vi "Frames.Initialize.vi"(6 "Direction":T1(ring), 8 "error in":errorcluster, 9 "Lookup":variant, 10 "Frames":T2[](array[typedef]) {"Signals"."Byte Order" items=["Little Endian", "Big Endian"]; "Signals"."Data Type" items=["Signed", "Unsigned", "IEEE Float"]}, 11 "Cluster In":refnum<k21>) -> (0 "error out":errorcluster, 1 "Lookup":variant, 3 "Cluster Out":refnum<k21>)   [LabVIEW 2019, in "Diagnostics Addon Engine.lvlib"]
uses:
  Diagnostics Addon Engine.lvlib
  Addon Shared/Types/Frame.Compile.ctl
  Addon Shared/Types/Type.ctl
  Addon Shared/Types/Signal.ctl
  Addon Shared/Types/XNET.Frame.ctl
  Addon Shared/SubVIs/Constants.vi
  <vilib>/xnet/xnet.llb/XNET Create Session (Conversion).vi
  Addon Shared/Diagnostics Addon Shared.lvlib
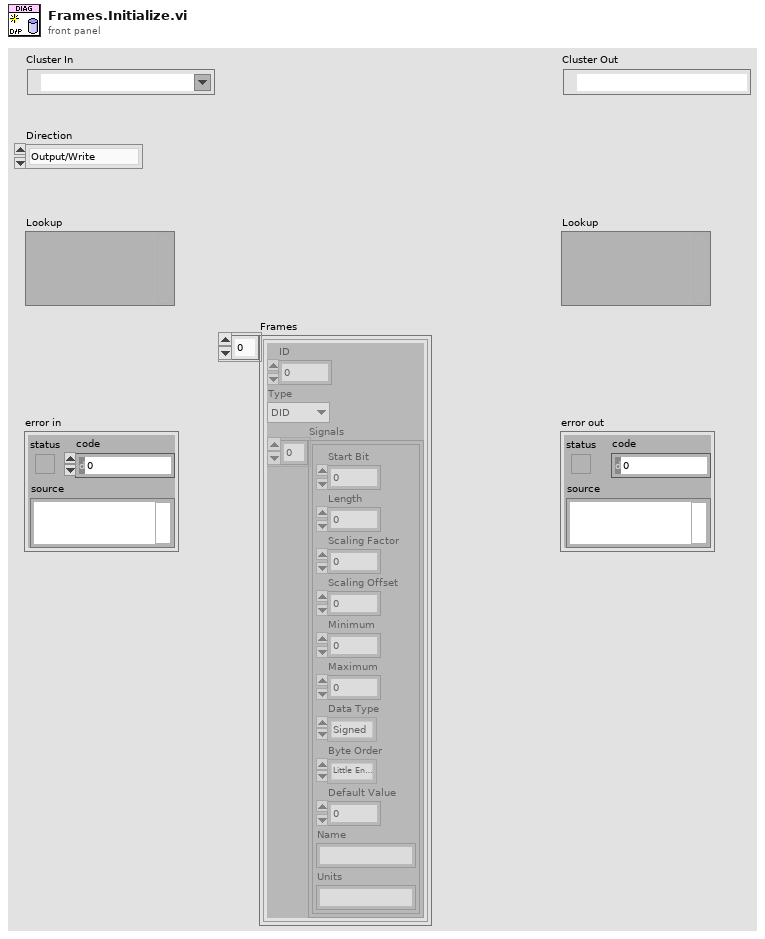
[diagram p1: front panel]
types:
  T1 = enum16{"Output/Write", "Input/Read", "Input/ReadWrite"}
  T2 = typedef "Diagnostics Addon Shared.lvlib/Frame.Compile.ctl" = cluster{"ID":u32, "Type":T3, "Signals":T4[]}
  T3 = typedef "Diagnostics Addon Shared.lvlib/Type.ctl" = enum16{"DID", "CDID", "PID", "CPID", "Read Memory", "Write Memory", "IO Control", "Routine Start", "Routine Request", "Routine Stop", "User Defined", "DTC Control", "Clear DTCs", "Read DTCs", "Start DTCs", "DTC Change Count", "Tester Present", "Unlock ECU", "Reset ECU", "Diag Session Control", "Communication Control", "DPID Control", "Poll Control", "Diag CAN Control"}
  T4 = typedef "Diagnostics Addon Shared.lvlib/Signal.ctl" = cluster{"Start Bit":u32, "Length":u32, "Scaling Factor":dbl, "Scaling Offset":dbl, "Minimum":dbl, "Maximum":dbl, "Data Type":u32, "Byte Order":u32, "Default Value":dbl, "Name":string, "Units":string}
  T5 = typedef "Diagnostics Addon Shared.lvlib/XNET.Frame.ctl" = cluster{"Frame name":string, "Identifier":u32, "Payload Length":u32, "Timing Type":u32, "Transmit Time":dbl, "Extended Identifier?":bool, "Comment":string, "IO Mode":u32}
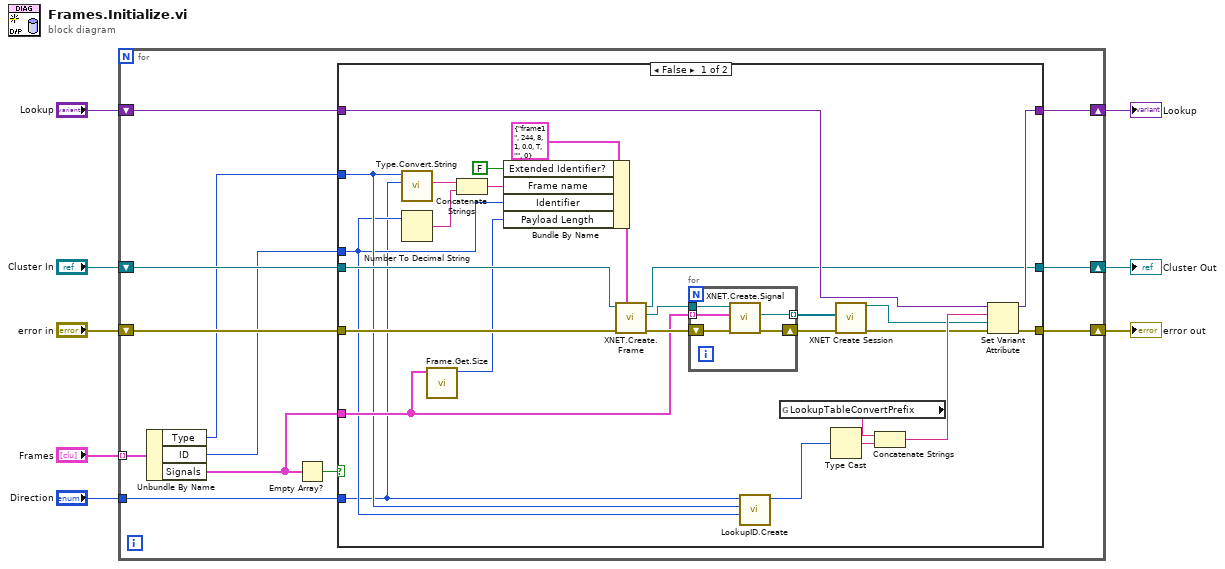
[diagram p0: block diagram]
diagram:
  n1 = for {
    shift-right: [w19] -> w7
    shift-left: "error in" -> [w16]
    tunnel: "Frames" -> [w20] mode=indexing
    shift-right: [w17] -> w5
    shift-left: "Lookup" -> [w18]
    shift-right: [w14] -> w2
    shift-left: "Cluster In" -> [w15]
    tunnel: "Direction" -> [w9]
    n2 = Unbundle By Name(w20) -> ("Type"=w12:T3, "ID"=w13:u32, "Signals"=w11:T4[])
    n3 = Empty Array?(array=w11) -> (empty?=w10:bool)
    n4 = case shown="False" w10 {
      tunnel: [w47 w55] -> w19
      tunnel: w18 -> [w46 w53]
      tunnel: [w45 w53] -> w17
      tunnel: w16 -> [w43 w55]
      tunnel: w15 -> [w38 w54]
      tunnel: [w36 w54] -> w14
      tunnel: w13 -> [w24 _]
      tunnel: w12 -> [w25 _]
      tunnel: w11 -> [w28 _]
      tunnel: w9 -> [w21 _]
      frame False {
        n5 = call "Type.Convert.String.vi"("Direction"=w21, "Type"=w25) -> ("ArbIDName"=w22:string)  [unwired: 8 in, 1 out]
        n6 = Number To Decimal String(number=w24) -> (decimal integer string=w35:string)  [unwired: 1 in]
        n7 = call "Frame.Get.Size.vi"("Parameters"=w28) -> ("Bytes"=w27:u32)  [unwired: 10 in]
        n8 = Concatenate Strings(w22, w35) -> (w41:string)
        n9 = Bundle By Name(cluster=T5 {"Frame name"="frame1", "Identifier"=244, "Payload Length"=8, "Timing Type"=1, "Transmit Time"=0.0, "Extended Identifier?"=TRUE, "Comment"="", "IO Mode"=0} ("CAN Frame"), "Extended Identifier?"=FALSE, "Frame name"=w41, "Identifier"=w24, "Payload Length"=w27) -> (w39:T5)
        n10 = call "XNET.Create.Frame.vi"("error in"=w43, "CAN Frame"=w39, "cluster in"=w38) -> ("error out"=w42:errorcluster, "frame out"=w37:refnum<k21>, "cluster out"=w36:refnum<k21>)  [unwired: 6 in]
        n11 = for {
          tunnel: w37 -> [w48]
          tunnel: w28 -> [w49] mode=indexing
          shift-right: [w51] -> w44
          shift-left: w42 -> [w52]
          tunnel: [w50] -> w34 mode=indexing
          n12 = call "XNET.Create.Signal.vi"("error in"=w52, "Signal"=w49, "frame in"=w48) -> ("error out"=w51:errorcluster, "signal out"=w50:refnum<k21>)  [unwired: 6 in, 1 out]
        }
        n13 = call "LookupID.Create.vi"("Serivce ID"=w24, "Service Type"=w25, "Direction"=w21) -> ("Result"=w23:u64)  [unwired: 8 in]
        n14 = global read "Constants.vi" "LookupTableConvertPrefix"() -> (w33:string)
        n15 = Type Cast(x=w23) -> (*(type *) &x=w29:string)  [unwired: 1 in]
        n16 = call-poly <vilib>:"XNET Create Session.vi"("signal list"=w34, "error in (no error)"=w44) -> ("session out"=w30:refnum<k21>, "error out"=w31:errorcluster)  [unwired: 1 in, 11 out]
        n17 = Concatenate Strings(w33, w29) -> (w32:string)
        n18 = Set Variant Attribute(Variant=w46, name=w32, value=w30, error in=w31) -> (Variant out=w45:variant, error out=w47:errorcluster)  [unwired: 1 out]
      }
      frame True {
      }
    }
  }
  "error out" <- w7
  "Cluster Out" <- w2
  "Lookup" <- w5
